vi "Read Temperature.vi"(7 "Initialize":bool, 8 "error in (no error)":errorcluster, 10 "Current Temperature":dbl, 11 "Freezer in":refnum<class "Freezer.lvclass">) -> (0 "error out":errorcluster, 1 "dT/dt":dbl, 2 "dT/dt - Lower":dbl, 3 "Freezer out":refnum<class "Freezer.lvclass">, 4 "T - Low Temp":dbl, 5 "T":dbl)   [LabVIEW 2015, in "cRIO-Carbondioxide.lvlib" / "CO2-Actor.lvlib" / "Freezer.lvclass"]
uses:
  Freezer.lvclass
  Freezer.lvclass/Freezer.ctl
  <vilib>/ptbypt/NI_PtbyPt.lvlib
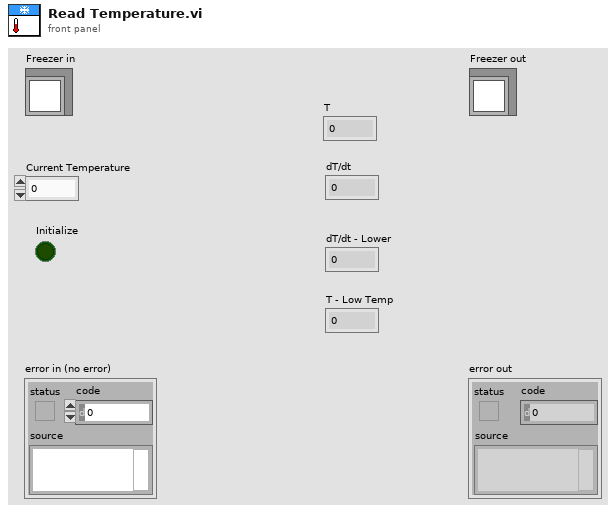
[diagram p1: front panel]
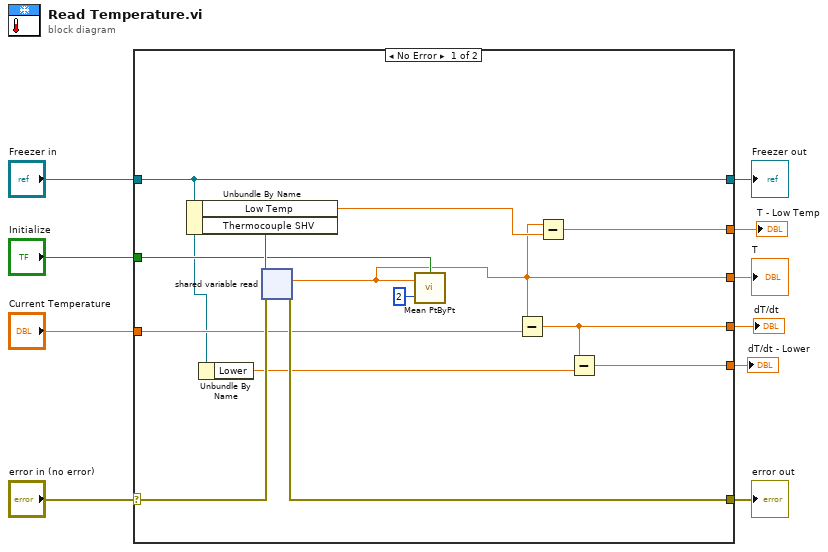
[diagram p0: block diagram]
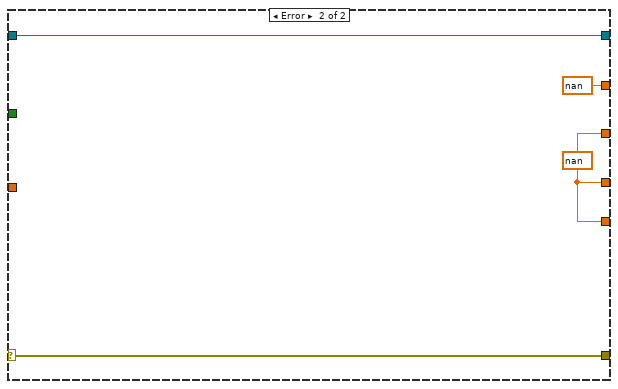
[diagram p2: hidden frame]
diagram:
  n1 = case shown="No Error" "error in (no error)" {
    selector: "error in (no error)" -> [w22 w27]
    tunnel: [w21 w27] -> w9
    tunnel: [w12 w26] -> w7
    tunnel: "Freezer in" -> [w12 w26]
    tunnel: [w11 w24] -> w6
    tunnel: "Initialize" -> [w19 _]
    tunnel: "Current Temperature" -> [w14 _]
    tunnel: [w17 w24] -> w3
    tunnel: [w18 nan] -> w2
    tunnel: [w15 w24] -> w1
    frame No Error {
      n2 = Unbundle By Name(w12) -> ("Low Temp"=w13:dbl, "Thermocouple SHV"=w23:refnum<k21>)
      n3 = Unbundle By Name(w12) -> ("Lower"=w16:dbl)
      n4 = shared-variable-read(w23, w22) -> (w21:errorcluster, w11:dbl)  [unwired: 2 out]
      n5 = call <vilib>:"Mean PtByPt.vi"("x"=w11, "sample length"=2, "initialize"=w19) -> ()  [unwired: 1 in, 2 out]
      n6 = Subtract(x=w11, y=w14) -> (x-y=w17:dbl)
      n7 = Subtract(x=w11, y=w13) -> (x-y=w18:dbl)
      n8 = Subtract(x=w17, y=w16) -> (x-y=w15:dbl)
    }
    frame Error {
      w24 = nan ("Syringe TC")
    }
  }
  "error out" <- w9
  "Freezer out" <- w7
  "T" <- w6
  "dT/dt" <- w3
  "T - Low Temp" <- w2
  "dT/dt - Lower" <- w1
